vi "resetSettledCheck.vi"(8 "error in (no error)":errorcluster, 11 "Model in":refnum<class "Model.lvclass">) -> (0 "error out":errorcluster, 2 "settledIsTrue":bool, 3 "Model out":refnum<class "Model.lvclass">)   [LabVIEW 2015, in "Model.lvclass"]
uses:
  Model.lvclass
  Model.lvclass/Model.ctl
  <userlib>/Common/ILC/ILC/ILC.lvclass/ILC.ctl
  ApplicationElements/SystemController/SystemController.lvclass
  <userlib>/Common/ILC/ILC/ILC.lvclass
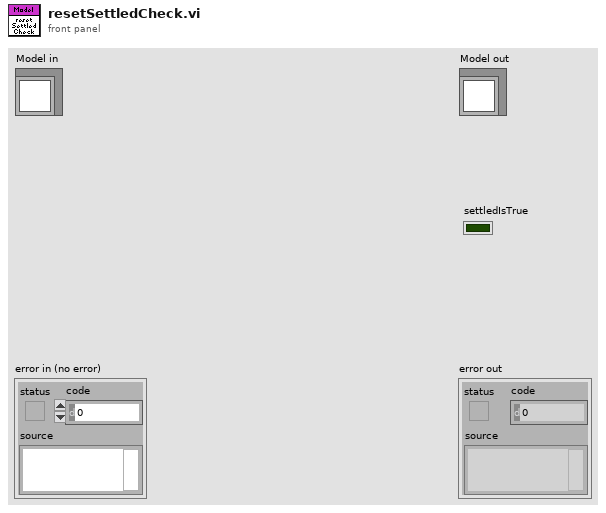
[diagram p1: front panel]
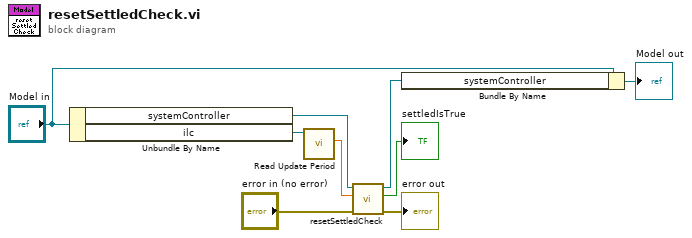
[diagram p0: block diagram]
diagram:
  n1 = Unbundle By Name("Model in") -> ("systemController"=w8:refnum<class "SystemController.lvclass">, "ilc"=w6:refnum<class "ILC.lvclass">)
  n2 = call <userlib>:"Read Update Period.vi"("ILC in"=w6) -> ("Update Period"=w5:dbl[unit])  [unwired: 9 in, 1 out]
  n3 = call "resetSettledCheck.vi"("error in (no error)"="error in (no error)", "loopPeriod"=w5, "SystemController in"=w8) -> ("error out"=→"error out":errorcluster, "settledIsTrue"=→"settledIsTrue":bool, "SystemController out"=w7:refnum<class "SystemController.lvclass">)  [unwired: 6 in]
  n4 = Bundle By Name(cluster="Model in", "systemController"=w7) -> (→"Model out":refnum<class "Model.lvclass">)
